vi "DAQmx Create Channel (CI-Pulse Time).vi"(0 "task in":refnum<k21>, 1 "maximum value":dbl=0.001 format="%.6f", 2 "minimum value":dbl=1e-06 format="%.6f", 5 "counter":tag, 7 "name to assign":string, 9 "units":i32(ring)=10364 items=["Seconds"=10364], 11 "error in":errorcluster) -> (4 "task out":refnum<k21>, 15 "error out":errorcluster)   [LabVIEW 2018]
doc: "Creates a channel to measure pulse specifications, returning the measurements as pairs of high time and low time. With the exception of devices that support multi-counter tasks, you can create only one counter input channel at a time with this VI because a task can contain only one counter input channel. To read from multiple counters simultaneously, use a separate task for each counter. Connect the input signal to the default input terminal of the counter unless you select a different input terminal."
uses:
  nilvaiu.dll
panel:
  # "input limits"
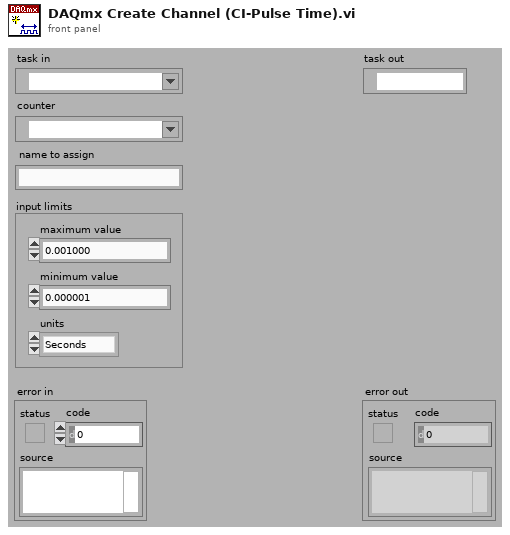
[diagram p1: front panel]
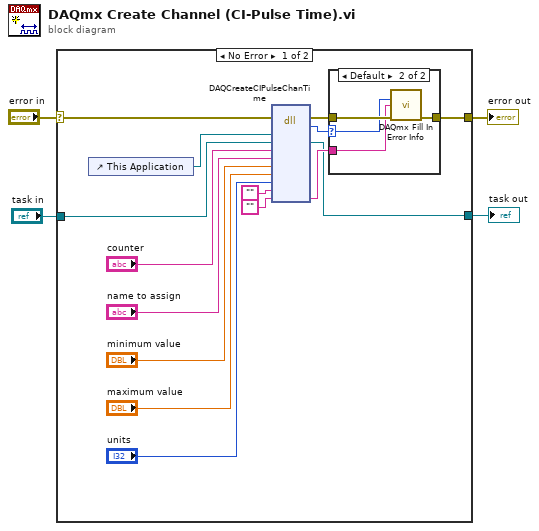
[diagram p0: block diagram]
diagram:
  n1 = case shown="No Error" "error in" {
    selector: "error in" -> [w6 w26]
    tunnel: [w9 w26] -> w4
    tunnel: [w8 w25] -> w3
    tunnel: "task in" -> [w7 w25]
    frame No Error {
      n2 = control-ref of="This Application"() -> (w16:refnum<vi>)
      n3 = dll-call lib="nilvaiu.*" fn="DAQCreateCIPulseChanTime"(error in=w6, "lvAppRef"=w16, "refObjPtr"=w7, "counter"="counter", "channelNameIn"="name to assign", "minVal"="minimum value", "maxVal"="maximum value", "units"="units", "channelNamesOut"="", "extendedErrorInfo"="") -> (error out=w19:errorcluster, "return type"=w18:i32, "refObjPtr"=w8:refnum<k21>, "extendedErrorInfo"=w17:string)  [unwired: 9 in, 1 out]
      n4 = case shown="Default" w18 {
        selector: w18 -> [_ w22]
        tunnel: w19 -> [w20 w24]
        tunnel: [w20 w23] -> w9
        tunnel: w17 -> [_ w21]
        frame 0 {
        }
        frame Default {
          n5 = call "DAQmx Fill In Error Info.vi"("status code"=w22, "extended error info"=w21, "error in"=w24) -> ("error out"=w23:errorcluster)  [unwired: 1 in, 11 out]
        }
      }
    }
    frame Error {
    }
  }
  "error out" <- w4
  "task out" <- w3
